vi "Agilent 34401A--Read voltage.vi"(2 "error in (no error)":errorcluster, 3 "Byte Count (1024 bytes)":i32=1024, 4 "34401A address":i16) -> (0 "error out":errorcluster, 1 "Numeric":dbl)   [LabVIEW 2013]
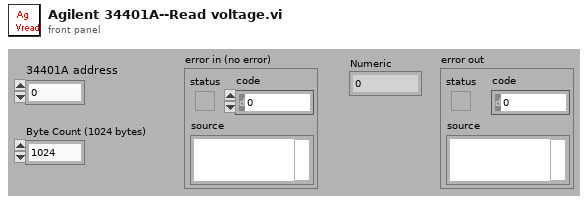
[diagram p1: front panel]
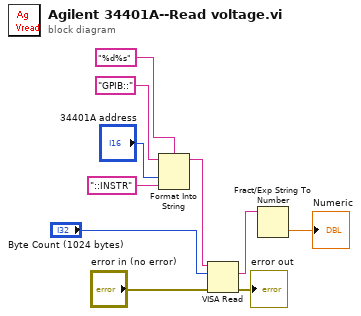
[diagram p0: block diagram]
diagram:
  n1 = Format Into String(format string="%d%s", initial string="GPIB::", "34401A address", "::INSTR" ("input 2")) -> (resulting string=w5:string)  [unwired: 1 in, 1 out]
  n2 = VISA Read(VISA resource name=w5, byte count="Byte Count (1024 bytes)", error in (no error)="error in (no error)") -> (read buffer=w4:string, error out=→"error out":errorcluster)  [unwired: 2 out]
  n3 = Fract/Exp String To Number(string=w4) -> (number=→"Numeric":dbl)  [unwired: 3 in, 1 out]
